vi "Software Reference Path Anchor.vi"() -> (3 "Reference Directory Path: Software":path)   [LabVIEW 2019]
doc: "This VI is used to identify an absolute reference path (often the software root directory) of a software system. This VI simply returns the path of the folder in which it is stored.\n\n(c) Copyright 1999, Alliance Technologies Group, Inc. This VI may not be duplicated, sold, or distributed without written consent from Alliance Technologies Group.JSMA Project Wizard 0.2.0.11\nRob Humfeld - JET Engineering\nCopyright (c) 2020, JET Engineering"
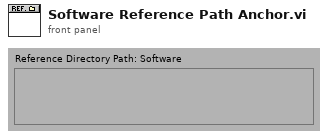
[diagram p1: front panel]
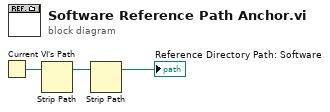
[diagram p0: block diagram]
diagram:
  n1 = Current VI's Path() -> (path=w3:path)
  n2 = Strip Path(path=w3) -> (stripped path=w2:path)  [unwired: 1 out]
  n3 = Strip Path(path=w2) -> (stripped path=→"Reference Directory Path: Software":path)  [unwired: 1 out]
